vi "GlobalInit.vi"(1 "错误输入（无错误）":errorcluster) -> (0 "错误输出":errorcluster)   [LabVIEW 2018]
uses:
  globalMessage.vi
  Reslut.vi
panel:
  out "实时消息":T1
  # "功率计"
  # "能量计"
  # "时间波形"
  # "光谱"
  # "偏振"
  # "近远场"
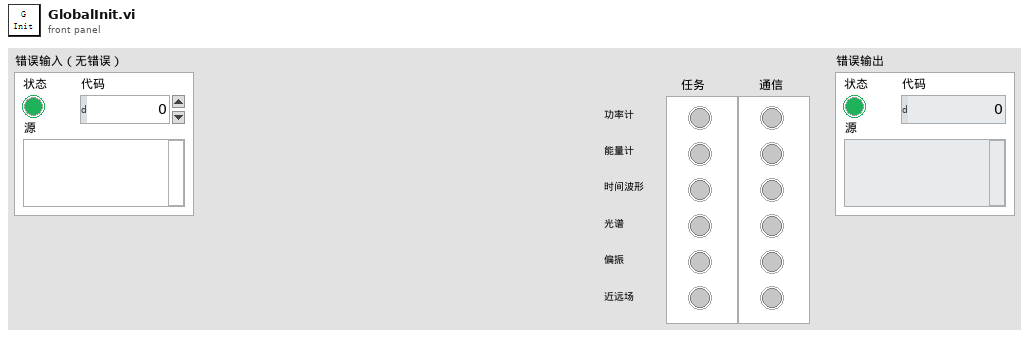
[diagram p1: front panel]
types:
  T1 = cluster{"任务":cluster{"功率任务":bool, "能量任务":bool, "时间波形任务":bool, "光谱任务":bool, "偏振任务":bool, "近远场任务":bool}, "通信":cluster{"功率通信":bool, "能量通信":bool, "时间波形通信":bool, "光谱通信":bool, "偏振通信":bool, "近远场通信":bool}}
  T2 = cluster{"能量计结果":string, "功率计结果":string, " 偏振方向":string, "偏振度":string}
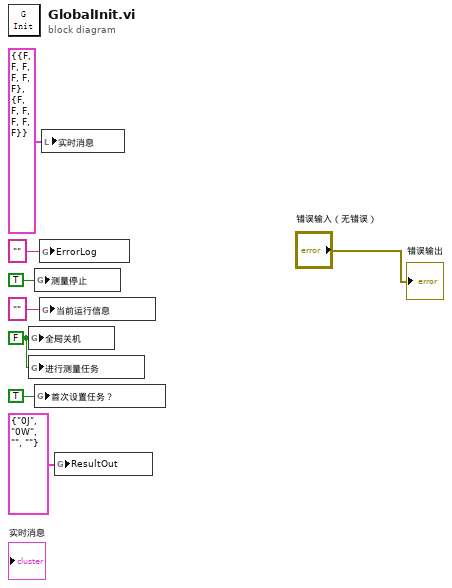
[diagram p0: block diagram]
diagram:
  w2 = FALSE ("全局关机")
  n1 = global write "参数.vi" "全局关机"(w2) -> ()
  n2 = global write "参数.vi" "进行测量任务"(w2) -> ()
  n3 = global write "参数.vi" "测量停止"(TRUE ("测量停止")) -> ()
  n4 = global write "globalMessage.vi" "首次设置任务？"(TRUE ("首次设置任务？")) -> ()
  n5 = global write "参数.vi" "ErrorLog"("" ("ErrorLog")) -> ()
  n6 = global write "globalMessage.vi" "当前运行信息"("" ("当前运行信息")) -> ()
  n7 = local write "实时消息"(T1 {"任务"={"功率任务"=FALSE, "能量任务"=FALSE, "时间波形任务"=FALSE, "光谱任务"=FALSE, "偏振任务"=FALSE, "近远场任务"=FALSE}, "通信"={"功率通信"=FALSE, "能量通信"=FALSE, "时间波形通信"=FALSE, "光谱通信"=FALSE, "偏振通信"=FALSE, "近远场通信"=FALSE}} ("实时消息")) -> ()
  n8 = global write "Reslut.vi" "ResultOut"(T2 {"能量计结果"="0J", "功率计结果"="0W", " 偏振方向"="", "偏振度"=""} ("ResultOut")) -> ()
  "错误输出" <- "错误输入（无错误）"
